vi "Teleportation.vi"   [LabVIEW 2020]
uses:
  QuSim/QuVI_Wire (initial).vi
  QuSim/QuVI_Wire (added).vi
  Analysis/Inspect VIs/Bloch Sphere - Display.vi
  Gates/Polymorphs/vControl_e.vi
  Gates/Polymorphs/Pauli-X_t.vi
  Gates/Polymorphs/Pauli-Z_s.vi
  Gates/Polymorphs/Pauli-X_s.vi
panel:
  # "Quantum Teleportation Example"
  # "*Open the block diagram for the circuit view (Ctrl+E)"
  # "Simulates the teleportation of an arbitrary qubit state from Alice to Bob.\n\nThis VI illustrates hybrid quantum-classical control. It uses a shared Bell pair to transfer a qubit's state. Note the green classical wires carrying measurement results from Alice; these drive Case Structures that apply conditional X and Z corrections to Bob's qubit, demonstrating the 'Classical Channel' requirement."
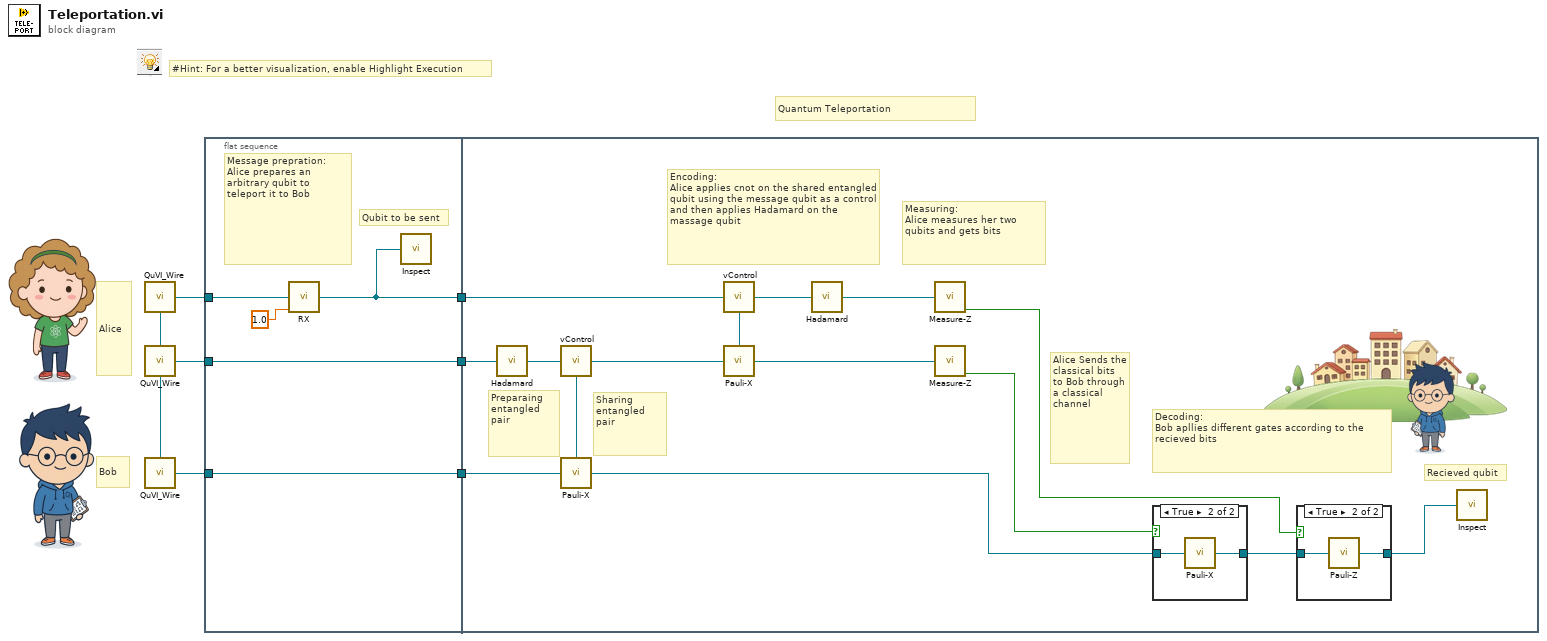
[diagram p0: block diagram]
diagram:
  # "#Hint: For a better visualization, enable Highlight Execution"
  # "Quantum Teleportation"
  # "Bob"
  # "Alice"
  n1 = call-poly "QuVI_Wire.vi"() -> ("QuWire out"=w8:refnum<class "QuWire.lvclass">, "Stack out"=w7:refnum<class "QuSim.lvclass">)  [unwired: 14 in]
  n2 = call-poly "QuVI_Wire.vi"("Stack in"=w7) -> ("QuWire out"=w5:refnum<class "QuWire.lvclass">, "Stack out"=w6:refnum<class "QuSim.lvclass">)  [unwired: 13 in]
  n3 = call-poly "QuVI_Wire.vi"("Stack in"=w6) -> ("QuWire out"=w4:refnum<class "QuWire.lvclass">)  [unwired: 13 in, 1 out]
  n4 = flat-sequence {
    tunnel: w4 -> [w12]
    tunnel: w5 -> [w13]
    tunnel: w8 -> [w9]
    tunnel: [w13] -> w3
    tunnel: [w12] -> w2
    tunnel: [w10] -> w1
    tunnel: w3 -> [w28]
    tunnel: w2 -> [w26]
    tunnel: w1 -> [w14]
    frame #0 {
      # "Qubit to be sent"
      # "Message prepration:\nAlice prepares an arbitrary qubit to teleport it to Bob"
      n5 = call "RX.vi"("QuWire in"=w9, "theta"=1.0) -> ("QuWire out"=w10:refnum<class "QuWire.lvclass">)  [unwired: 13 in]
      n6 = call-poly "Inspect.vi"("QuWire in"=w10) -> ()  [unwired: 15 in]
    }
    frame #1 {
      # "Recieved qubit"
      # "Sharing entangled pair"
      # "Preparaing entangled pair"
      # "Decoding:\nBob apllies different gates according to the recieved bits"
      # "Alice Sends the classical bits to Bob through a classical channel"
      # "Measuring:\nAlice measures her two qubits and gets bits"
      # "Encoding:\nAlice applies cnot on the shared entangled qubit using the message qubit as a control and then applies Hadamard on the massage qubit"
      n7 = call "Hadamard.vi"("QuWire in"=w28) -> ("QuWire out"=w27:refnum<class "QuWire.lvclass">)  [unwired: 14 in]
      n8 = call-poly "vControl.vi"("QuWire in"=w27) -> ("QuWire out"=w23:refnum<class "QuWire.lvclass">, "v Ctrl out"=w25:refnum<class "CtrlLine.lvclass">)  [unwired: 13 in]
      n9 = call-poly "Pauli-X.vi"("v Ctrl  in"=w25, "QuWire in"=w26) -> ("QuWire out"=w17:refnum<class "QuWire.lvclass">)  [unwired: 13 in]
      n10 = call-poly "vControl.vi"("QuWire in"=w14) -> ("QuWire out"=w22:refnum<class "QuWire.lvclass">, "v Ctrl out"=w24:refnum<class "CtrlLine.lvclass">)  [unwired: 13 in]
      n11 = call-poly "Pauli-X.vi"("v Ctrl  in"=w24, "QuWire in"=w23) -> ("QuWire out"=w21:refnum<class "QuWire.lvclass">)  [unwired: 13 in]
      n12 = call "Hadamard.vi"("QuWire in"=w22) -> ("QuWire out"=w20:refnum<class "QuWire.lvclass">)  [unwired: 14 in]
      n13 = call "Measure-Z.vi"("QuWire in"=w20) -> ("Classical bit"=w19:bool)  [unwired: 13 in, 1 out]
      n14 = call "Measure-Z.vi"("QuWire in"=w21) -> ("Classical bit"=w18:bool)  [unwired: 13 in, 1 out]
      n15 = case shown="True" w18 {
        tunnel: w17 -> [w32 w34]
        tunnel: [w32 w33] -> w16
        frame False {
        }
        frame True {
          n16 = call-poly "Pauli-X.vi"("QuWire in"=w34) -> ("QuWire out"=w33:refnum<class "QuWire.lvclass">)  [unwired: 14 in]
        }
      }
      n17 = case shown="True" w19 {
        tunnel: w16 -> [w29 w31]
        tunnel: [w29 w30] -> w15
        frame False {
        }
        frame True {
          n18 = call-poly "Pauli-Z.vi"("QuWire in"=w31) -> ("QuWire out"=w30:refnum<class "QuWire.lvclass">)  [unwired: 14 in]
        }
      }
      n19 = call-poly "Inspect.vi"("QuWire in"=w15) -> ()  [unwired: 15 in]
    }
  }
